vi "Extract GPIO Data from Timestamps.vi"(0 "gpio timestamps in":T2[](array[typedef]), 5 "max samples to preallocate":i32=1000000, 7 "max gpio bank":T1=enum."Ser0 GPIO Bank", 9 "min gpio bank":T1=enum."Ser0 GPIO Bank", 11 "seconds to add to end for display":dbl=0.5 format="%#_13g") -> (4 "gpio timestamps out":T4(array[cluster]))   [LabVIEW 2023, in "GettingStarted_Common_148X_Host.lvlib"]
uses:
  GettingStarted_Common_148X_Host.lvlib
  <instrlib>/FlexRIO/CSI-2/v2/Host/Types/Host GPIO Bank Timestamp.ctl
  <instrlib>/FlexRIO/CSI-2/v2/FPGA/Types/Timestamp ID.ctl
  <instrlib>/FlexRIO/CSI-2/v2/FPGA/Types/GPIO Bank.ctl
  Types/GPIO Format Data.ctl
  <instrlib>/FlexRIO/CSI-2/v2/FPGA/NI CSI-2 API FPGA v2.lvlib
  <instrlib>/FlexRIO/CSI-2/v2/Host/NI CSI-2 API Host v2.lvlib
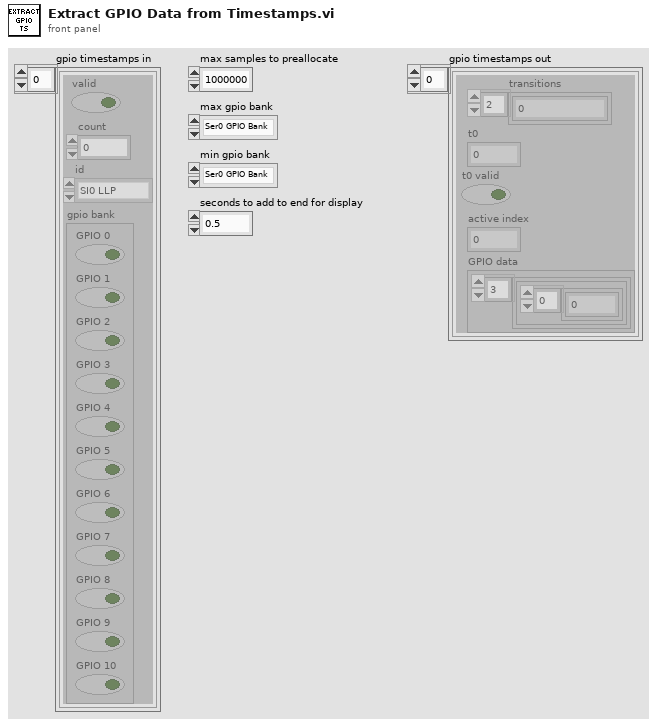
[diagram p1: front panel]
types:
  T1 = typedef "NI CSI-2 API FPGA v2.lvlib/Timestamp ID.ctl" = enum8{"SI0 LLP", "SI1 LLP", "SI2 LLP", "SI3 LLP", "SI4 LLP", "SI5 LLP", "SI6 LLP", "SI7 LLP", "SO0 LLP", "SO1 LLP", "SO2 LLP", "SO3 LLP", "SO4 LLP", "SO5 LLP", "SO6 LLP", "SO7 LLP", "Ser0 GPIO Bank", "Ser1 GPIO Bank", "Ser2 GPIO Bank", "Ser3 GPIO Bank", "Ser4 GPIO Bank", "Ser5 GPIO Bank", "Ser6 GPIO Bank", "Ser7 GPIO Bank", "Des0 GPIO Bank", "Des1 GPIO Bank", "Des2 GPIO Bank", "Des3 GPIO Bank", "Des4 GPIO Bank", "Des5 GPIO Bank", "Des6 GPIO Bank", "Des7 GPIO Bank", "User0", "User1", "User2", "User3", "User4", "User5", "User6", "User7", "User8", "User9", "User10", "User11", "User12", "User13", "User14", "User15", "User16", "User17", "User18", "User19", "User20", "User21", "User22", "User23", "User24", "User25", "User26", "User27", "User28", "User29", "User30", "User31"}
  T2 = typedef "NI CSI-2 API Host v2.lvlib/Host GPIO Bank Timestamp.ctl" = cluster{"valid":bool, "count":u64, "id":T1, "gpio bank":T3}
  T3 = typedef "NI CSI-2 API FPGA v2.lvlib/GPIO Bank.ctl" = cluster{"GPIO 0":bool, "GPIO 1":bool, "GPIO 2":bool, "GPIO 3":bool, "GPIO 4":bool, "GPIO 5":bool, "GPIO 6":bool, "GPIO 7":bool, "GPIO 8":bool, "GPIO 9":bool, "GPIO 10":bool}
  T4 = cluster{"transitions":u64[], "t0":u64, "t0 valid":bool, "active index":i32, "GPIO data":cluster{cluster{u8[]}[]}}[]
  T5 = typedef "GettingStarted_Common_148X_Host.lvlib/GPIO Format Data.ctl" = cluster{"transitions":u64[], "t0":u64, "t0 valid":bool, "active index":i32, "GPIO data":cluster{cluster{u8[]}[]}}
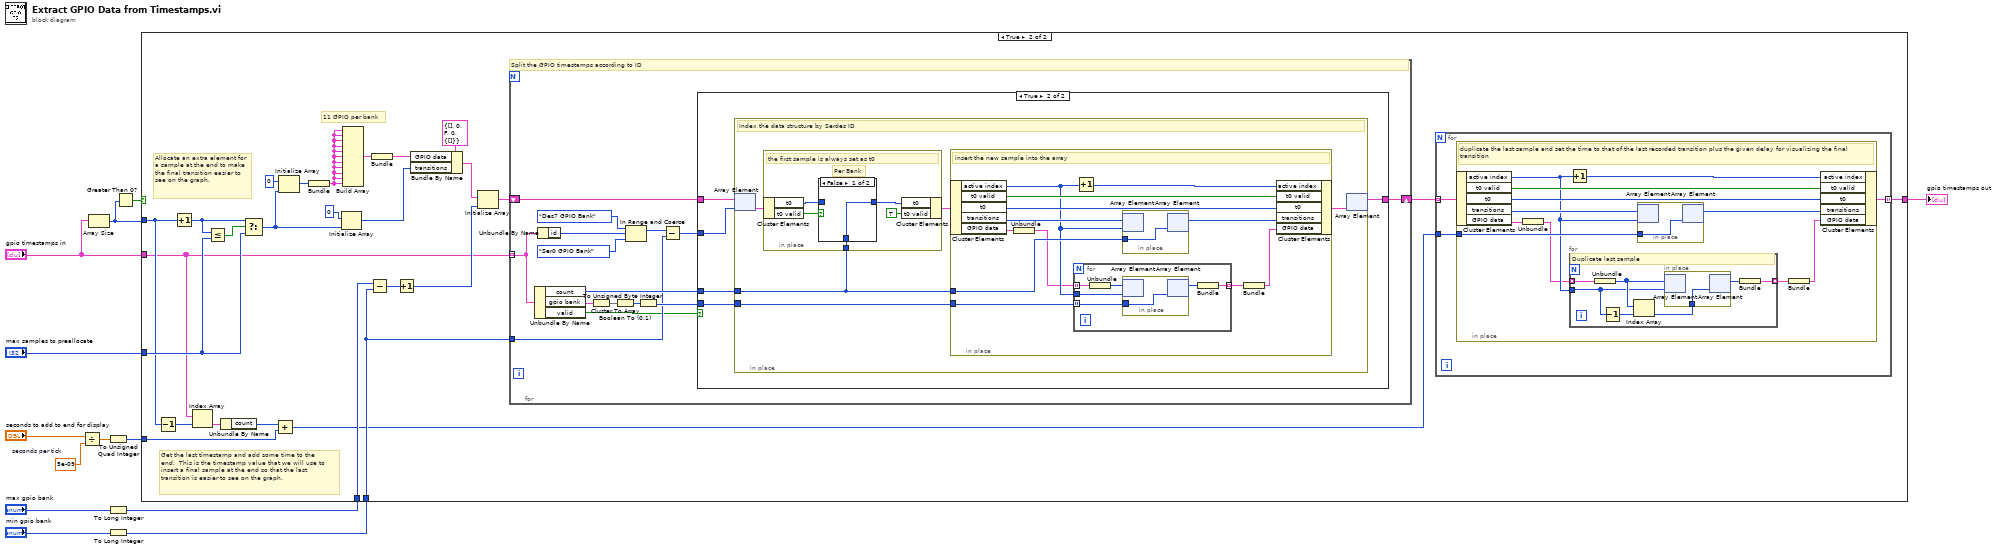
[diagram p0: block diagram]
diagram:
  w6 = 5e-09  # seconds per tick
  n1 = Divide(x="seconds to add to end for display", y=w6) -> (x/y=w4:dbl)
  n2 = Array Size(array="gpio timestamps in") -> (size(s)=w12:i32)
  n3 = To Unsigned Quad Integer(1:w4) -> (0:w3:u64)
  n4 = To Long Integer(number="max gpio bank") -> (32bit integer=w2:i32)
  n5 = To Long Integer(number="min gpio bank") -> (32bit integer=w1:i32)
  n6 = Greater Than 0?(x=w12) -> (x > 0?=w7:bool)
  n7 = case shown="True" w7 {
    tunnel: "gpio timestamps in" -> [_ w22]
    tunnel: [_ w18] -> w13
    tunnel: w1 -> [_ w35]
    tunnel: w2 -> [_ w36]
    tunnel: w12 -> [_ w23]
    tunnel: "max samples to preallocate" -> [_ w27]
    tunnel: w3 -> [_ w21]
    frame False {
    }
    frame True {
      # "Allocate an extra element for a sample at the end to make the final transition easier to see on the graph."
      # "Get the last timestamp and add some time to the end.  This is the timestamp value that we will use to insert a final sample at the end so that the last transition is easier to see on the graph."
      # "11 GPIO per bank"
      n8 = Decrement(x=w23) -> (x-1=w16:i32)
      n9 = Increment(x=w23) -> (x+1=w20:i32)
      n10 = Index Array(array=w22, index=w16) -> (element=w15:T2)
      n11 = Less Or Equal?(x=w20, y=w27) -> (x <= y?=w33:bool)
      n12 = Unbundle By Name(w15) -> ("count"=w14:u64)
      n13 = Select(t=w20, s=w33, f=w27) -> (s? t:f=w24:i32)
      n14 = Add(x=w14, y=w21) -> (x+y=w17:u64)
      n15 = Initialize Array(u8 0, w24) -> (w31:u8[])
      n16 = Bundle(w31) -> (w30:cluster{u8[]})  [unwired: 1 in]
      n17 = Initialize Array(u64 0, w24) -> (w38:u64[])
      n18 = Build Array(w30, w30, w30, w30, w30, w30, w30, w30, w30, w30, w30) -> (w28:cluster{u8[]}[])
      n19 = Subtract(x=w36, y=w35) -> (x-y=w34:i32)
      n20 = Bundle(w28) -> (w26:cluster{cluster{u8[]}[]})  [unwired: 1 in]
      n21 = Increment(x=w34) -> (x+1=w25:i32)
      n22 = Bundle By Name(cluster=T5 {"transitions"=[], "t0"=0, "t0 valid"=FALSE, "active index"=0, "GPIO data"={[]}}, "GPIO data"=w26, "transitions"=w38) -> (w29:T5)
      n23 = Initialize Array(w29, w25) -> (w40:T5[])
      n24 = for {
        tunnel: w22 -> [w47] mode=indexing
        shift-right: [w45] -> w19
        shift-left: w40 -> [w46]
        tunnel: w35 -> [w43]
        # "Split the GPIO timestamps according to ID"
        n25 = Unbundle By Name(w47) -> ("count"=w44:u64, "gpio bank"=w49:T3, "valid"=w42:bool)
        n26 = Unbundle By Name(w47) -> ("id"=w52:T1)
        n27 = Cluster To Array(cluster=w49) -> (array=w50:bool[])
        n28 = Boolean To (0,1)(Boolean=w50) -> (0, 1=w51:i16[])
        n29 = In Range and Coerce(upper limit=Timestamp_ID."Des7 GPIO Bank" ("y"), x=w52, lower limit=Timestamp_ID."Ser0 GPIO Bank" ("y")) -> (coerced(x)=w55:T1)  [unwired: 1 out]
        n30 = To Unsigned Byte Integer(number=w51) -> (unsigned 8bit integer=w48:u8[])
        n31 = Subtract(x=w55, y=w43) -> (x-y=w41:i32)
        n32 = case shown="True" w42 {
          tunnel: w48 -> [_ w61]
          tunnel: w46 -> [w56 w60]
          tunnel: [w56 w59] -> w45
          tunnel: w44 -> [_ w58]
          tunnel: w41 -> [_ w57]
          frame False {
            # "Don't count transitions on invalid timestamps"
          }
          frame True {
            n33 = in-place {
              in-place-border: w58 -> [w62]
              in-place-border: w61 -> [w66]
              # "Index the data structure by Serdes ID"
              n34 = in-place-array #1(w60, w57) -> (w65:T5)
              n35 = in-place {
                in-place-border: w62 -> [w68]
                # "Per Bank"
                # "the first sample is always set as t0"
                n36 = in-place-cluster #2(w65) -> ("t0"=w69:u64, "t0 valid"=w71:bool)
                n37 = case shown="False" w71 {
                  tunnel: [w72 w73] -> w70
                  tunnel: w69 -> [_ w73]
                  tunnel: w68 -> [w72 _]
                  frame False {
                  }
                  frame True {
                  }
                }
                n38 = in-place-cluster #2("t0"=w70, "t0 valid"=TRUE) -> (w64:T5)
              }
              n39 = in-place {
                in-place-border: w66 -> [w78]
                in-place-border: w62 -> [w82]
                # "insert the new sample into the array"
                n40 = in-place-cluster #3(w64) -> ("active index"=w79:i32, "t0 valid"=w81:bool, "t0"=w80:u64, "transitions"=w85:u64[], "GPIO data"=w75:cluster{cluster{u8[]}[]})
                n41 = Unbundle(w75) -> (w77:cluster{u8[]}[])
                n42 = for {
                  tunnel: [w91] -> w76 mode=indexing
                  tunnel: w77 -> [w90] mode=indexing
                  tunnel: w79 -> [w87]
                  tunnel: w78 -> [w86] mode=indexing
                  n43 = Unbundle(w90) -> (w89:u8[])
                  n44 = in-place {
                    in-place-border: w86 -> [w92]
                    n45 = in-place-array #4(w89, w87) -> ()  [unwired: 1 out]
                    n46 = in-place-array #4(w92) -> (w88:u8[])  [unwired: 1 out]
                  }
                  n47 = Bundle(w88) -> (w91:cluster{u8[]})  [unwired: 1 in]
                }
                n48 = Increment(x=w79) -> (x+1=w84:i32)
                n49 = in-place {
                  in-place-border: w82 -> [w93]
                  n50 = in-place-array #5(w85, w79) -> ()  [unwired: 1 out]
                  n51 = in-place-array #5(w93) -> (w83:u64[])  [unwired: 1 out]
                }
                n52 = Bundle(w76) -> (w74:cluster{cluster{u8[]}[]})  [unwired: 1 in]
                n53 = in-place-cluster #3("active index"=w84, "t0 valid"=w81, "t0"=w80, "transitions"=w83, "GPIO data"=w74) -> (w63:T5)
              }
              n54 = in-place-array #1(w63) -> (w59:T5[])  [unwired: 1 out]
            }
          }
        }
      }
      n55 = for {
        tunnel: w19 -> [w96] mode=indexing
        tunnel: [w94] -> w18 mode=indexing
        tunnel: w17 -> [w95]
        n56 = in-place {
          in-place-border: w95 -> [w104]
          # "duplicate the last sample and set the time to that of the last recorded transition plus the given delay for visualizing the final transition"
          n57 = in-place-cluster #6(w96) -> ("active index"=w101:i32, "t0 valid"=w103:bool, "t0"=w102:u64, "transitions"=w107:u64[], "GPIO data"=w98:cluster{cluster{u8[]}[]})
          n58 = Unbundle(w98) -> (w100:cluster{u8[]}[])
          n59 = Increment(x=w101) -> (x+1=w106:i32)
          n60 = for {
            tunnel: [w114] -> w99 mode=indexing
            tunnel: w100 -> [w113] mode=indexing
            tunnel: w101 -> [w109]
            # "Duplicate last sample"
            n61 = Unbundle(w113) -> (w111:u8[])
            n62 = Decrement(x=w109) -> (x-1=w108:i32)
            n63 = Index Array(array=w111, index=w108) -> (element=w110:u8)
            n64 = in-place {
              in-place-border: w110 -> [w115]
              n65 = in-place-array #7(w111, w109) -> ()  [unwired: 1 out]
              n66 = in-place-array #7(w115) -> (w112:u8[])  [unwired: 1 out]
            }
            n67 = Bundle(w112) -> (w114:cluster{u8[]})  [unwired: 1 in]
          }
          n68 = in-place {
            in-place-border: w104 -> [w116]
            n69 = in-place-array #8(w107, w101) -> ()  [unwired: 1 out]
            n70 = in-place-array #8(w116) -> (w105:u64[])  [unwired: 1 out]
          }
          n71 = Bundle(w99) -> (w97:cluster{cluster{u8[]}[]})  [unwired: 1 in]
          n72 = in-place-cluster #6("active index"=w106, "t0 valid"=w103, "t0"=w102, "transitions"=w105, "GPIO data"=w97) -> (w94:T5)
        }
      }
    }
  }
  "gpio timestamps out" <- w13
